vi "subvi_cluster_Axsun.vi"(4 "wave length":dbl, 5 "output cluster in in":T1, 6 "LaserONTime":dbl, 7 "device array":string[](array[string]), 9 "String":string, 10 "Numeric":i32, 11 "control version":string) -> (3 "output cluster in out":T1)   [LabVIEW 2018]
uses:
  Control 2.ctl
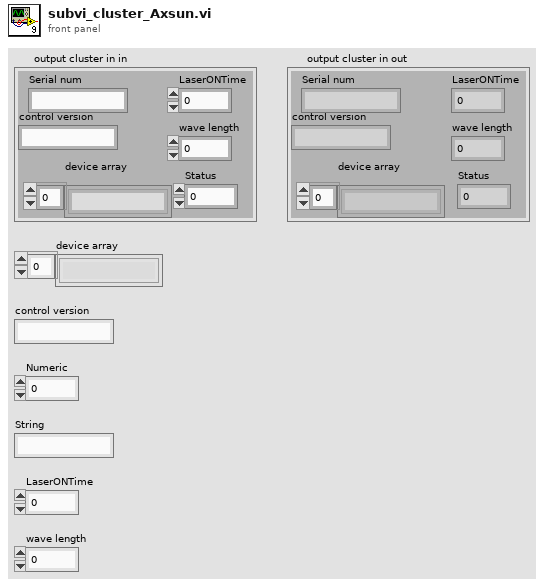
[diagram p1: front panel]
types:
  T1 = typedef "Control 2.ctl" = cluster{"device array":string[], "control version":string, "Serial num":string, "LaserONTime":i32, "wave length":dbl, "Status":dbl}
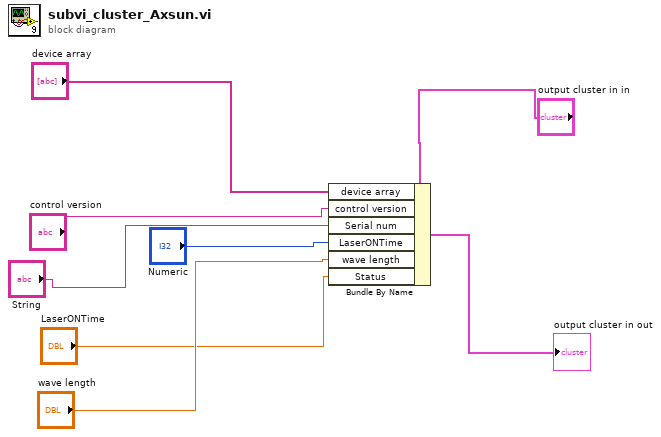
[diagram p0: block diagram]
diagram:
  n1 = Bundle By Name(cluster="output cluster in in", "device array"="device array", "control version"="control version", "Serial num"="String", "LaserONTime"="Numeric", "wave length"="wave length", "Status"="LaserONTime") -> (→"output cluster in out":T1)
